vi "Intake Mode Select.vi"(10 "Manual":bool, 11 "Auto":bool) -> (3 "Intake Mode":T1)   [LabVIEW 2016]
uses:
  Common Code/Intake Mode.ctl
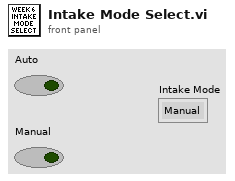
[diagram p1: front panel]
types:
  T1 = typedef "Intake Mode.ctl" = enum16{"Manual", "Auto"}
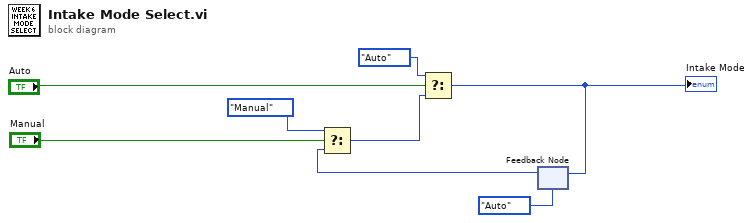
[diagram p0: block diagram]
diagram:
  n1 = feedback #1(Intake_Mode."Auto" ("Intake Mode")) -> (w1:T1)
  n2 = Select(t=Intake_Mode."Manual" ("Intake Mode"), s="Manual", f=w1) -> (s? t:f=w4:T1)
  n3 = Select(t=Intake_Mode."Auto" ("Intake Mode"), s="Auto", f=w4) -> (s? t:f=w2:T1)
  "Intake Mode" <- w2
  n4 = feedback-in #1(w2) -> ()
